vi "System@UserPanelCMD__Parameter.vi"(1 "ParamterIn":string) -> (0 "ParamterOut":string)   [LabVIEW 2020]
panel:
  in  "Parameters":string(combo)
  in  "VI":string(combo)
  in  "Confirm":bool
  # "System@UserPanelCMD $CMD,$Parameter"
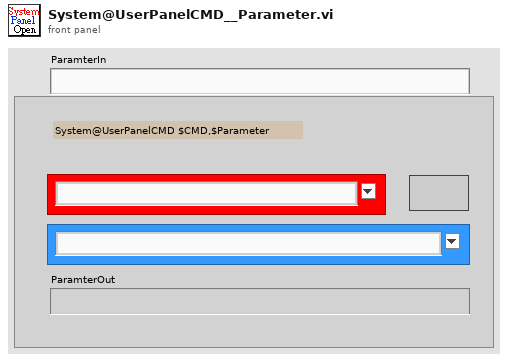
[diagram p1: front panel]
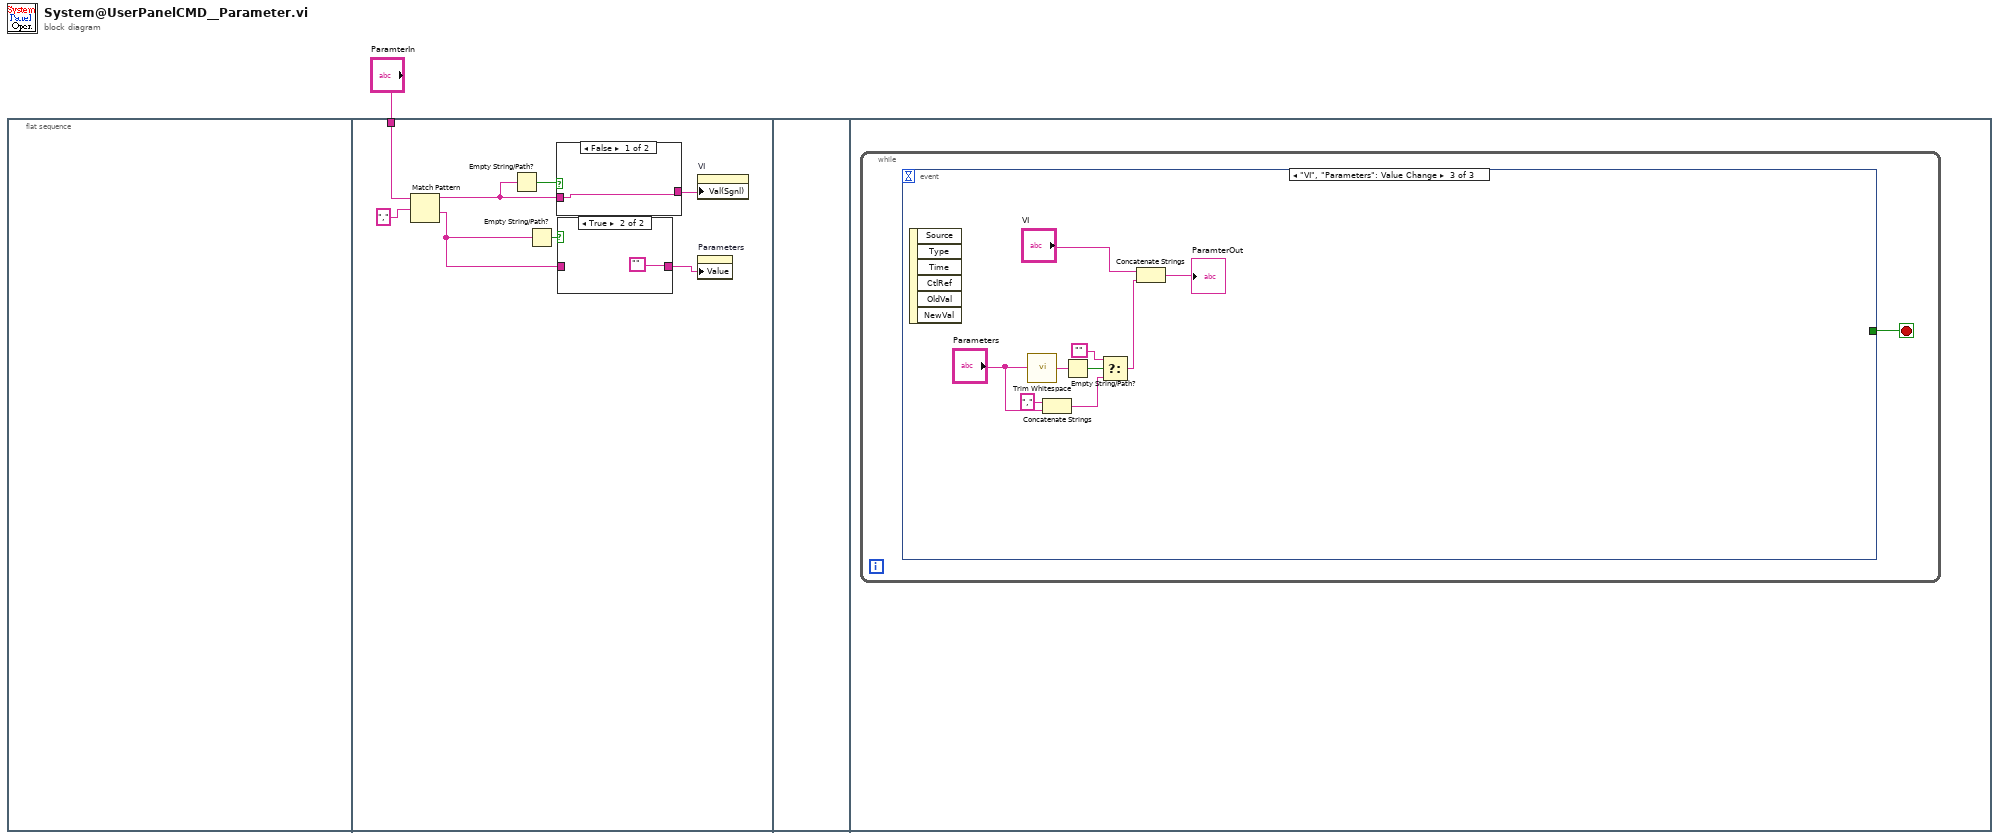
[diagram p0: block diagram]
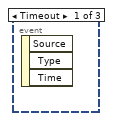
[diagram p4: hidden frame]
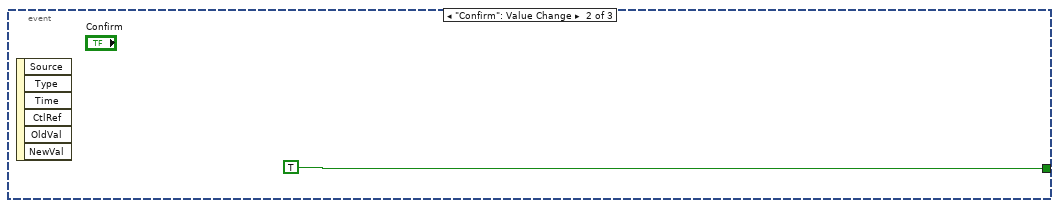
[diagram p5: hidden frame]
diagram:
  n1 = flat-sequence {
    tunnel: "ParamterIn" -> [w7]
    frame #0 {
    }
    frame #1 {
      n2 = Match Pattern(string=w7, regular expression=",") -> (before substring=w5:string, after substring=w4:string)  [unwired: 1 in, 2 out]
      n3 = Empty String/Path?(string/path=w5) -> (empty?=w9:bool)
      n4 = Empty String/Path?(string/path=w4) -> (empty?=w8:bool)
      n5 = case shown="False" w9 {
        tunnel: w5 -> [w12 w13]
        tunnel: [w12 w13] -> w2
        frame False {
        }
        frame True {
        }
      }
      n6 = case shown="True" w8 {
        tunnel: [w10 ""] -> w3
        tunnel: w4 -> [w10 _]
        frame False {
        }
        frame True {
        }
      }
      n7 = property on="VI" class="CmbBox"("Val(Sgnl)"=w2) -> ()  [unwired: 2 in, 2 out]
      n8 = property on="Parameters" class="CmbBox"("Value"=w3) -> ()  [unwired: 2 in, 2 out]
    }
    frame #2 {
    }
    frame #3 {
      n9 = while {
        stop <- w14 stop-if-true
        n10 = event shown="[2] \"VI\", \"Parameters\": Value Change" {
          selector: _ -> [_ _ _]
          dyn-events: _ -> [_ _ _]
          timeout: _ -> [_ _ _]
          tunnel: [_ TRUE _] -> w14
          event Timeout {
            n11 = event-data() -> ()  [unwired: 1 in, 3 out]
          }
          event "Confirm": Value Change {
            n12 = event-data() -> ()  [unwired: 1 in, 6 out]
          }
          event "VI", "Parameters": Value Change {
            n13 = event-data() -> ()  [unwired: 1 in, 6 out]
            n14 = call <vilib>:"Trim Whitespace.vi"("string"="Parameters") -> ("trimmed string"=w21:string)  [unwired: 1 in]
            n15 = Concatenate Strings("," ("string"), "Parameters") -> (w20:string)
            n16 = Empty String/Path?(string/path=w21) -> (empty?=w22:bool)
            n17 = Select(t="", s=w22, f=w20) -> (s? t:f=w17:string)
            n18 = Concatenate Strings("VI", w17) -> (→"ParamterOut":string)
          }
        }
      }
    }
  }
